vi "test.vi"() -> ()   [LabVIEW 2018]
panel:
  in  "Y Scale":enum16{"nanoAmps", "microAmps", "milliAmps"}(ring)
  out "Data":cluster{dbl[], dbl[], dbl[], dbl[], dbl[]}[](array[cluster])
  out "Re-Generated":cluster{dbl[], dbl[]}[](graph)
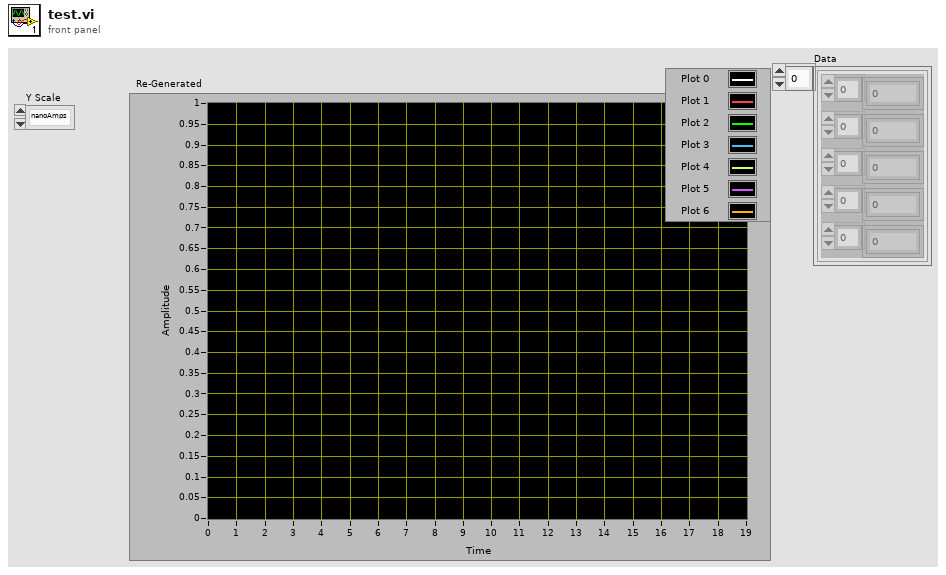
[diagram p1: front panel]
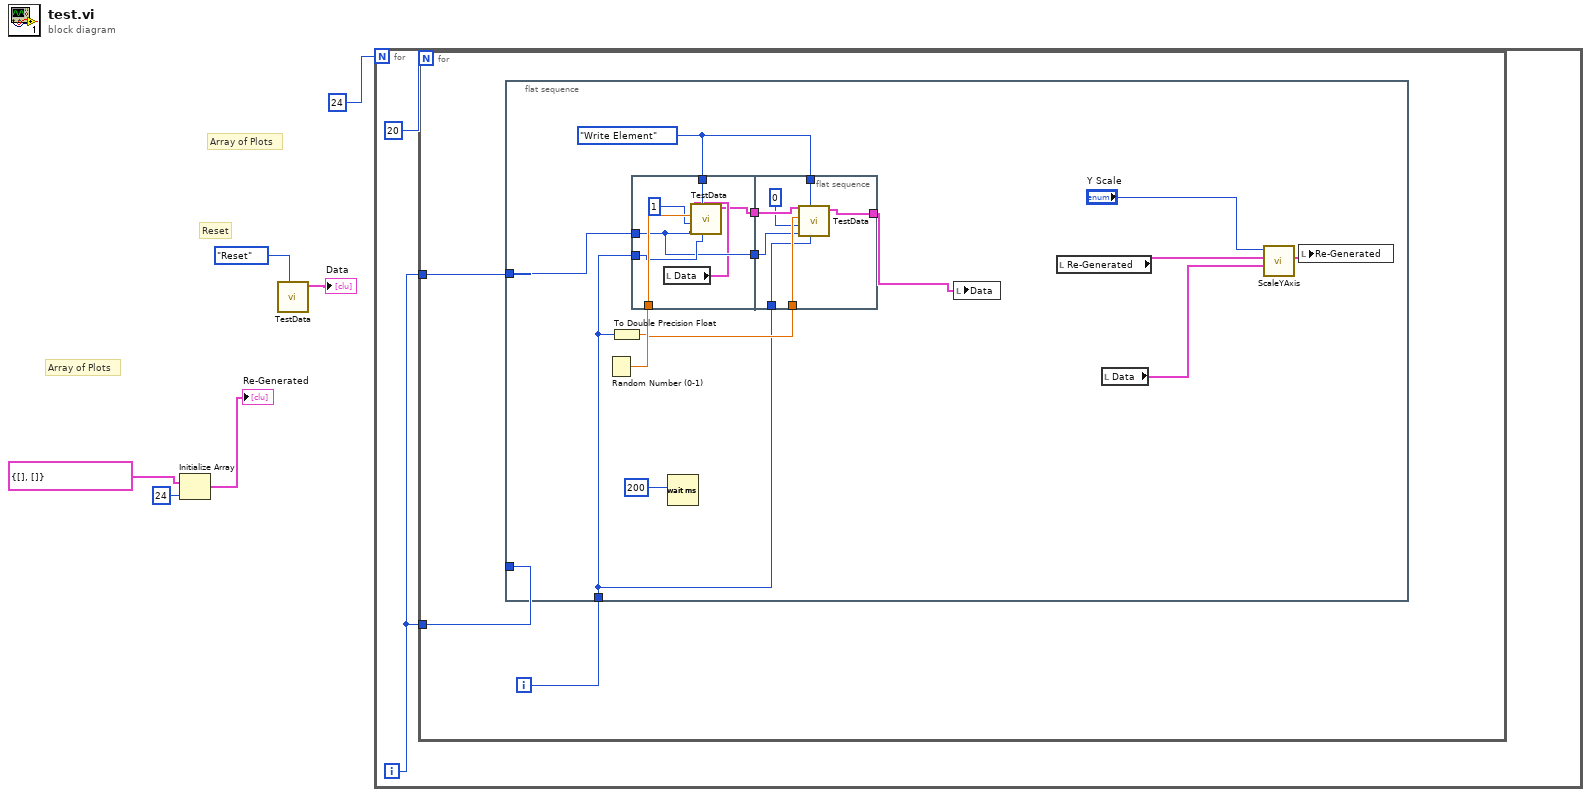
[diagram p0: block diagram]
diagram:
  # "Array of Plots"
  # "Reset"
  # "Array of Plots"
  n1 = Initialize Array(cluster{dbl[], dbl[]} {[], []}, 24 ("dimension size")) -> (→"Re-Generated":cluster{dbl[], dbl[]}[])
  n2 = call "TestData.vi"("Action"=enum16{"Reset", "Write Element", "Read Array"}."Reset") -> ("Data OUT"=→"Data":cluster{dbl[], dbl[], dbl[], dbl[], dbl[]}[])  [unwired: 9 in, 1 out]
  n3 = for {
    N: 24 -> [_]
    i -> [w7]
    n4 = for {
      N: 20 -> [_]
      tunnel: w7 -> [w10]
      tunnel: w7 -> [w9]
      i -> [w11]
      n5 = flat-sequence {
        tunnel: w11 -> [w18]
        tunnel: w10 -> [w21]
        tunnel: w9 -> [_]
        frame #0 {
          w19 = enum16{"Reset", "Write Element", "Read Array"}."Write Element" ("Action")
          n6 = Random Number (0-1)() -> (number: 0 to 1=w24:dbl)
          n7 = To Double Precision Float(number=w18) -> (double precision float=w22:dbl)
          n8 = flat-sequence {
            tunnel: w24 -> [w31]
            tunnel: w18 -> [w29]
            tunnel: w21 -> [w28]
            tunnel: [w28] -> w20
            tunnel: w19 -> [w30]
            tunnel: [w25] -> w16
            tunnel: [w38] -> w17
            tunnel: w22 -> [w37]
            tunnel: w18 -> [w35]
            tunnel: w20 -> [w34]
            tunnel: w19 -> [w36]
            tunnel: w16 -> [w33]
            frame #0 {
              n9 = local read "Data"() -> (w26:cluster{dbl[], dbl[], dbl[], dbl[], dbl[]}[])
              n10 = call "TestData.vi"("Reading No."=w29, "Action"=w30, "Test No."=w28, "Array No."=u32 1, 10:"Data IN"=w31, 11:"Data IN"=w26) -> ("Data OUT"=w25:cluster{dbl[], dbl[], dbl[], dbl[], dbl[]}[])  [unwired: 4 in, 1 out]
            }
            frame #1 {
              n11 = call "TestData.vi"("Reading No."=w35, "Action"=w36, "Test No."=w34, "Array No."=u32 0, 10:"Data IN"=w37, 11:"Data IN"=w33) -> ("Data OUT"=w38:cluster{dbl[], dbl[], dbl[], dbl[], dbl[]}[])  [unwired: 4 in, 1 out]
            }
          }
          n12 = Wait (ms)(milliseconds to wait=u32 200) -> ()  [unwired: 1 out]
          n13 = local write "Data"(w17) -> ()
          n14 = local read "Re-Generated"() -> (w13:cluster{dbl[], dbl[]}[])
          n15 = local read "Data"() -> (w14:cluster{dbl[], dbl[], dbl[], dbl[], dbl[]}[])
          n16 = call "ScaleYAxis.vi"("Data IN"=w14, "Plot In"=w13, "Y Scale"="Y Scale") -> ("Plot Out"=w15:cluster{dbl[], dbl[]}[])  [unwired: 8 in]
          n17 = local write "Re-Generated"(w15) -> ()
        }
      }
    }
  }
